vi "CFTS-Get Postexposure Time.vi"(0 "Expt State":T1, 11 "error in (no error)":errorcluster) -> (8 "Postexposure Time (min)":dbl, 15 "error out":errorcluster)   [LabVIEW 2020]
uses:
  CFTS-Experiment State.ctl
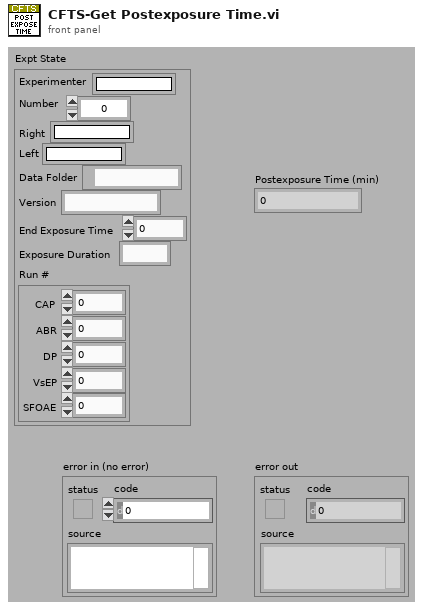
[diagram p1: front panel]
types:
  T1 = typedef "CFTS-Experiment State.ctl" = cluster{"Experimenter":string, "Number":u32, "Right":string, "Left":string, "Data Folder":path, "Version":string, "End Exposure Time":dbl, "Exposure Duration":string, "Run #":cluster{"CAP":i32, "ABR":i32, "DP":i32, "VsEP":i32, "SFOAE":i32}}
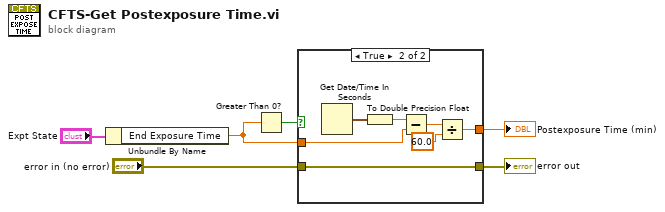
[diagram p0: block diagram]
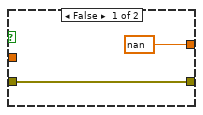
[diagram p2: hidden frame]
diagram:
  n1 = Unbundle By Name("Expt State") -> ("End Exposure Time"=w2:dbl)
  n2 = Greater Than 0?(x=w2) -> (x > 0?=w6:bool)
  n3 = case shown="True" w6 {
    tunnel: w2 -> [_ w13]
    tunnel: [nan w10] -> w5
    tunnel: "error in (no error)" -> [w7 w9]
    tunnel: [w7 w9] -> w4
    frame False {
    }
    frame True {
      n4 = Get Date/Time In Seconds() -> (seconds since 1Jan1904=w15:timestamp)
      n5 = To Double Precision Float(number=w15) -> (double precision float=w14:dbl)
      n6 = Subtract(x=w14, y=w13) -> (x-y=w12:dbl)
      n7 = Divide(x=w12, y=60.0) -> (x/y=w10:dbl)
    }
  }
  "error out" <- w4
  "Postexposure Time (min)" <- w5
